vi "Delete Class.vi"(8 "error in (no error)":errorcluster, 10 "Classes":refnum<class>[](array[class]), 11 "Tag Tree In":refnum<class "LVCLass Tree.lvclass">) -> (0 "error out":errorcluster, 3 "Tag Tree Out":refnum<class "LVCLass Tree.lvclass">)   [LabVIEW 2020, in "Tree Helpers.lvlib" / "LVCLass Tree.lvclass"]
uses:
  LVCLass Tree.lvclass
  LVCLass Tree.lvclass/LVCLass Tree.ctl
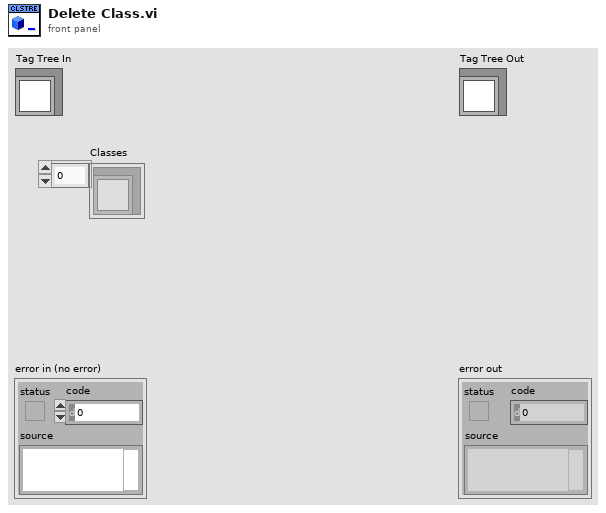
[diagram p1: front panel]
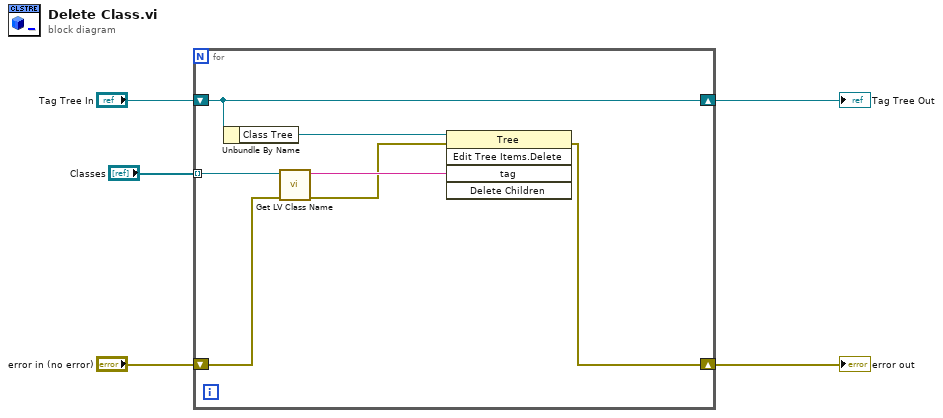
[diagram p0: block diagram]
diagram:
  n1 = for {
    tunnel: "Classes" -> [w8] mode=indexing
    shift-right: [w11] -> w2
    shift-left: "error in (no error)" -> [w6]
    shift-right: [w10] -> w1
    shift-left: "Tag Tree In" -> [w10]
    n2 = Unbundle By Name(w10) -> ("Class Tree"=w12:refnum<vi>)
    n3 = call <vilib>:"Get LV Class Name.vi"("error in (no error)"=w6, "object"=w8) -> ("error out"=w7:errorcluster, "class name"=w9:string)  [unwired: 8 in]
    n4 = invoke class="Tree" method="Edit Tree Items.Delete"(reference=w12, error in=w7, "tag"=w9) -> (error out=w11:errorcluster)  [unwired: 2 in, 4 out]
  }
  "error out" <- w2
  "Tag Tree Out" <- w1
